vi "CloseConnection.vi"(8 "error in (no error)":errorcluster, 10 "Connection Number":i32, 11 "TCP_Server in":refnum<class "TCP_Server.lvclass">) -> (0 "error out":errorcluster, 3 "TCP_Server out":refnum<class "TCP_Server.lvclass">)   [LabVIEW 2023, in "TCP_Server.lvlib" / "TCP_Server.lvclass"]
uses:
  TCP_Server.lvclass
  C:/Program Files (x86)/National Instruments/LabVIEW 2023/vi.lib/ActorFramework/Actor/Actor.lvclass
  <vilib>/ActorFramework/Actor/Actor.lvclass/Actor.ctl
  <vilib>/ActorFramework/Message Enqueuer/Message Enqueuer.lvclass/Message Enqueuer.ctl
  TCP_Server.lvclass/TCP_Server.ctl
  <vilib>/ActorFramework/Message Enqueuer/Init from Existing Queue.vi
  <vilib>/ActorFramework/Message Enqueuer/Enqueue.vi
  TCP_Server_Connection_Handler/TCP_Server_Connection_Handler Messages/CloseConnection Msg/CloseConnection Msg.lvclass
  C:/Program Files (x86)/National Instruments/LabVIEW 2023/vi.lib/ActorFramework/Message/Message.lvclass
  TCP_Server Messages/UpdateGUIconnectionTable Msg/UpdateGUIconnectionTable Msg.lvclass
  <vilib>/ActorFramework/Message Priority Queue/Priority Enqueue.vi
  <vilib>/ActorFramework/Message Enqueuer/Message Enqueuer.lvclass
  <vilib>/ActorFramework/Actor/Actor.lvclass
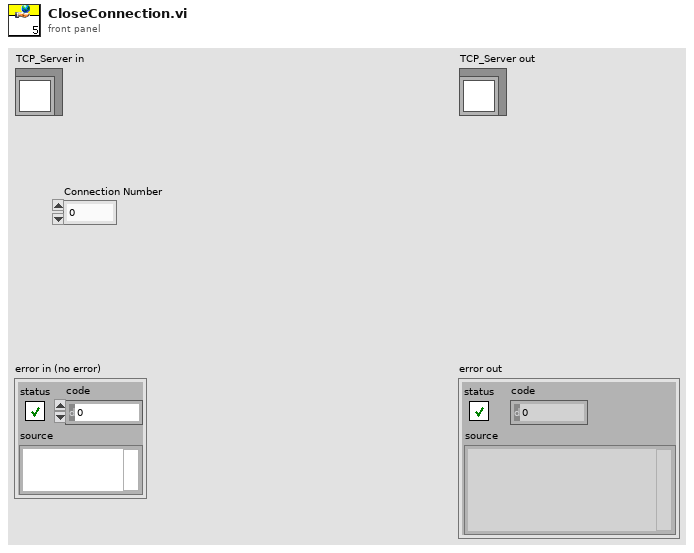
[diagram p1: front panel]
types:
  T1 = typedef "TCP_Server.lvlib/ServerConnection.ctl" = cluster{"Connection Handlers's Enqueuer":refnum<class "Message Enqueuer.lvclass">, "Connection Window's Enqueuer":refnum<class "Message Enqueuer.lvclass">, "Connection Information":T2}
  T2 = typedef "TCP_Listener.lvlib/ConnectionInformation.ctl" = cluster{"Connection number":i32, "Remote Address":string, "Remote Port":u16, "Connection ID":refnum<k5>}
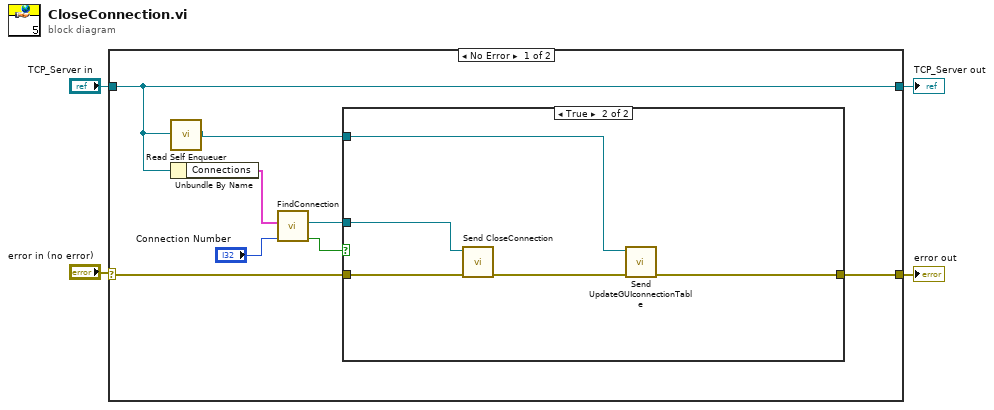
[diagram p0: block diagram]
diagram:
  n1 = case shown="No Error" "error in (no error)" {
    selector: "error in (no error)" -> [w9 w19]
    tunnel: "TCP_Server in" -> [w8 w20]
    tunnel: [w8 w20] -> w2
    tunnel: [w7 w19] -> w1
    frame No Error {
      n2 = call <vilib>:"Read Self Enqueuer.vi"("Actor"=w8) -> ("Self Enqueuer"=w6:refnum<class "Message Enqueuer.lvclass">)  [unwired: 10 in]
      n3 = Unbundle By Name(w8) -> ("Connections"=w12:T1[])
      n4 = call "FindConnection.vi"("Connection number"="Connection Number", "Connections"=w12) -> ("Found?"=w5:bool, "Connection Handlers's Enqueuer"=w10:refnum<class "Message Enqueuer.lvclass">)  [unwired: 6 in, 2 out]
      n5 = case shown="True" w5 {
        tunnel: w10 -> [_ w18]
        tunnel: w9 -> [w13 w17]
        tunnel: [w13 w15] -> w7
        tunnel: w6 -> [_ w14]
        frame False {
        }
        frame True {
          n6 = call "Send CloseConnection.vi"("error in (no error)"=w17, "Message Enqueuer"=w18) -> ("error out"=w16:errorcluster)  [unwired: 8 in, 1 out]
          n7 = call "Send UpdateGUIconnectionTable.vi"("error in (no error)"=w16, "Message Enqueuer"=w14) -> ("error out"=w15:errorcluster)  [unwired: 8 in, 1 out]
        }
      }
    }
    frame Error {
    }
  }
  "error out" <- w1
  "TCP_Server out" <- w2
